vi "main RT.vi"() -> ()   [LabVIEW 2020]
uses:
  <vilib>/Platform/TimedLoop/XDataNode/timing_clust.ctl
  <vilib>/Platform/TimedLoop/XDataNode/nitl_modes.ctl
  <vilib>/Platform/TimedLoop/XDataNode/wakeup.ctl
  <vilib>/Model Interface Toolkit/Model Interface Toolkit.lvclass/Model Interface Toolkit.ctl
  <vilib>/Model Interface Toolkit/Model Update.vi
  <vilib>/Model Interface Toolkit/Tick Model.vi
  <vilib>/Model Interface Toolkit/Probe Signals.vi
  <vilib>/Model Interface Toolkit/Multirate/Dispatch Model Tasks.vi
  <vilib>/Model Interface Toolkit/Call Model Start Routine.vi
  <vilib>/Model Interface Toolkit/Handle Error.vi
  <vilib>/Model Interface Toolkit/Multirate/Wait on Tasks.vi
  <vilib>/Model Interface Toolkit/Check Error.vi
  <vilib>/Model Interface Toolkit/Generate Error Cluster.vi
  <vilib>/Platform/TimedLoop/scheduler/LVUserAPI/Fire Software-Triggered Timing Source.vi
  <vilib>/Platform/TimedLoop/XDataNode/XDataNode.xnode
  <vilib>/Model Interface Toolkit/Model Interface Toolkit.lvclass
  <vilib>/Platform/TimedLoop/XDataNode/XDNodeRunTimeDep.lvlib
panel:
  out "Postition":dbl(graph)
  in  "Numeric":dbl
  out "Pressure":dbl(graph)
  out "Velocity":dbl(graph)
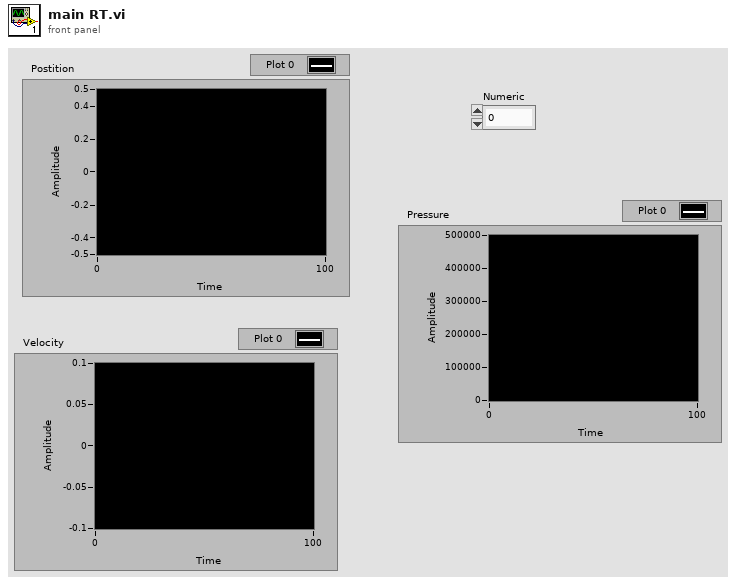
[diagram p1: front panel]
types:
  T1 = typedef "XDNodeRunTimeDep.lvlib/timing_clust.ctl" = cluster{"Expected End [f-1]":u64, "Actual End [f-1]":u64, "Finished Late? [f-1]":bool, "Expected End [i-1]":u64, "Actual End [i-1]":u64, "Finished Late? [i-1]":bool, "Expected Start [i]":u64, "Actual Start [i]":u64, "Expected Start [f]":u64, "Actual Start [f]":u64, "Source Name":string, "Structure Name":string, "Period":i64, "Deadline":i64, "Offset":i64, "Start":i64, "Priority":i32, "Timeout":i32, "Mode":T2, "Wakeup Reason":T3, "Error":errorcluster, "Source Type":string, "Secondary Source Type":string, "Global End Time":u64, "Global Start Time":u64, "Frame Duration":u64, "Iteration Duration":u64, "Assigned CPU":i32, "I/O Scan Engine Mode":u32}
  T2 = typedef "XDNodeRunTimeDep.lvlib/nitl_modes.ctl" = enum32{"No Change", "Process missed periods, maintain original phase", "Discard missed periods, maintain original phase", "Process missed periods, ignore original phase", "Discard missed periods, ignore original phase"}
  T3 = typedef "XDNodeRunTimeDep.lvlib/wakeup.ctl" = enum32{"Normal", "Aborted", "Asynchronous wakeup", "Timing source error", "Timed loop error", "Timeout"}
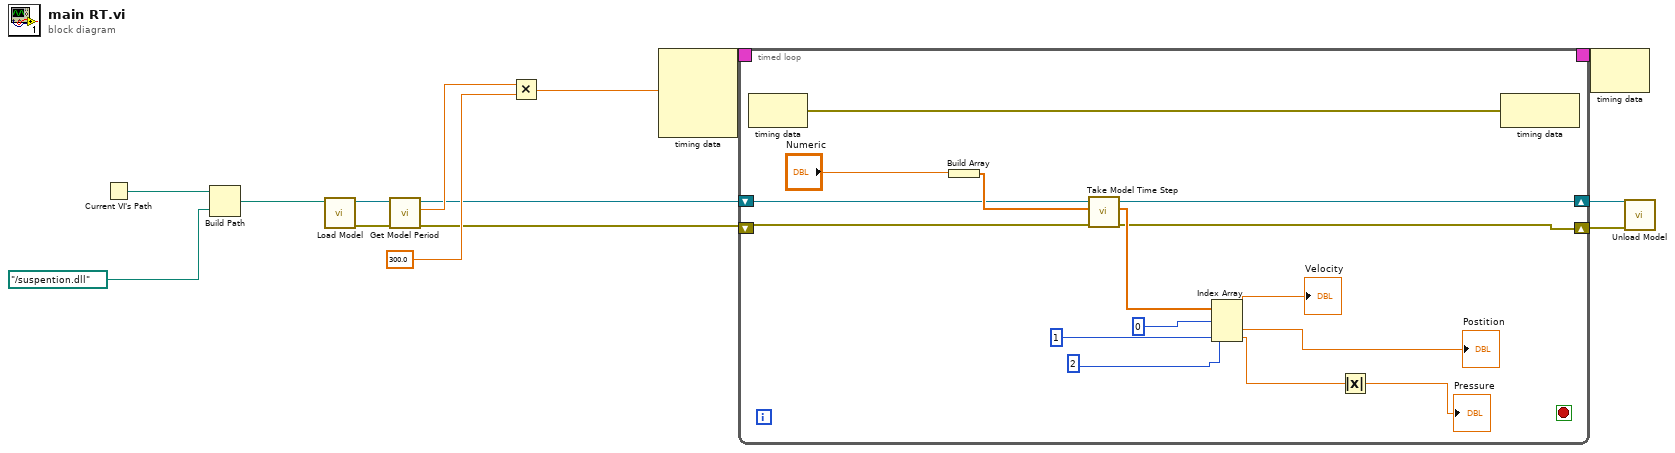
[diagram p0: block diagram]
diagram:
  n1 = Current VI's Path() -> (path=w8:path)
  n2 = Build Path(base path=w8, name or relative path=path "../suspention.dll" ("Model Path")) -> (appended path=w7:path)
  n3 = call <vilib>:"Load Model.vi"("Model Path"=w7) -> ("error out"=w11:errorcluster, "Model out"=w12:refnum<class "Model Interface Toolkit.lvclass">)  [unwired: 9 in]
  n4 = call <vilib>:"Get Model Period.vi"("error in"=w11, "Model in"=w12) -> ("error out"=w1:errorcluster, "Model Period (s)"=w10:dbl, "Model out"=w4:refnum<class "Model Interface Toolkit.lvclass">)  [unwired: 7 in]
  n5 = Multiply(x=w10, y=300.0) -> (x*y=w6:dbl)
  n6 = node-c288(w6) -> (w14:T1)  [unwired: 3 in]
  n7 = timed-loop {
    timing: w14 -> [_]
    timing-out: [_] -> w13
    shift-right: [w19] -> w3
    shift-left: w4 -> [w20]
    shift-right: [w18] -> w2
    shift-left: w1 -> [w17]
    stop <- _ stop-if-true
    n8 = node-c288() -> (w28:errorcluster)  [unwired: 1 in]
    n9 = Build Array("Numeric") -> (w29:dbl[])
    n10 = call <vilib>:"Take Model Time Step.vi"("error in (no error)"=w17, "Inport Array"=w29, "Model in"=w20) -> ("error out"=w18:errorcluster, "Outport Array out"=w27:dbl[], "Model out"=w19:refnum<class "Model Interface Toolkit.lvclass">)  [unwired: 6 in]
    n11 = Index Array(array=w27, index #1=0 ("index"), index #2=1 ("index"), index #3=2 ("index")) -> (element #1=→"Velocity":dbl, element #2=→"Postition":dbl, element #3=w16:dbl)
    n12 = Absolute Value(x=w16) -> (abs(x)=→"Pressure":dbl)
    n13 = node-c288(w28) -> ()  [unwired: 1 out]
  }
  n14 = node-c288(w13) -> ()  [unwired: 1 out]
  n15 = call <vilib>:"Unload Model.vi"("error in (no error)"=w2, "Model in"=w3) -> ()  [unwired: 9 in, 1 out]
